vi "BotSpeak_HTTP.vi"(0 "BotSpeak File Name":path, 1 "URL":string, 2 "BotSpeak Code":string, 3 "cookie file":path) -> (7 "connection\nerror":errorcluster, 8 "file error":errorcluster)   [LabVIEW 2014]
uses:
  <vilib>/httpClient/POSTFile.vi
  <vilib>/httpClient/LabVIEWHTTPClient.lvlib
panel:
  # "Macintosh HD:Users:gabbyvukasin:Documents:Tufts:Independent Study:EV3Server:BotSpeakCode.txt"
  # "Macintosh HD:Users:gabbyvukasin:Documents:Tufts:Independent Study:EV3Server:cookies.txt"
  # "SET DIO[1],1"
  # "192.168.2.3:2012"
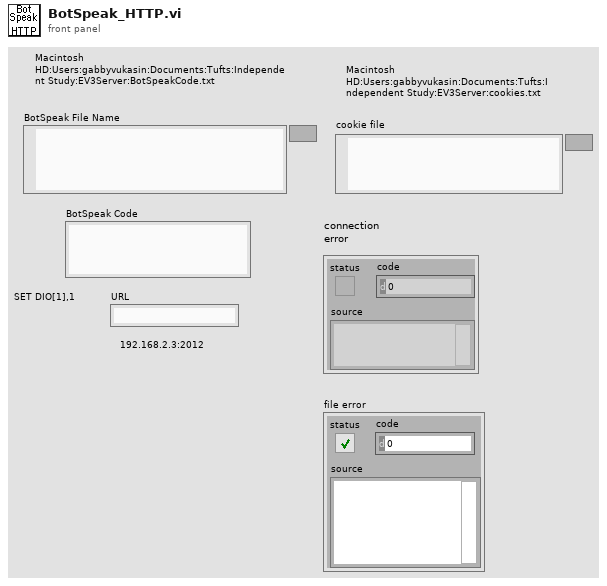
[diagram p1: front panel]
types:
  T1 = typedef "LabVIEWHTTPClient.lvlib/ClientHandle.ctl" = refnum<k1>
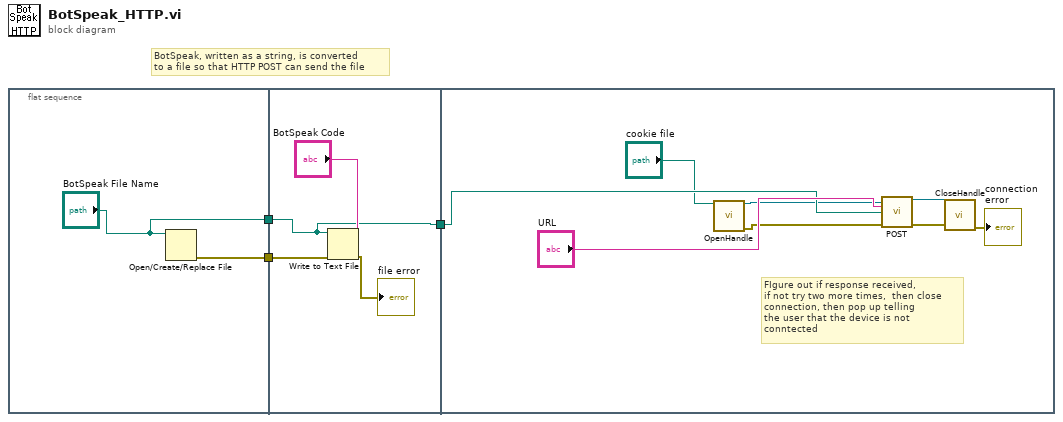
[diagram p0: block diagram]
diagram:
  # "BotSpeak, written as a string, is converted\nto a file so that HTTP POST can send the file"
  n1 = flat-sequence {
    tunnel: ["BotSpeak File Name"] -> w2
    tunnel: [w5] -> w1
    tunnel: [w6] -> w3
    tunnel: w2 -> [w6]
    tunnel: w1 -> [w8]
    tunnel: w3 -> [w14]
    frame #0 {
      n2 = Open/Create/Replace File(file path (use dialog)="BotSpeak File Name") -> (error out=w5:errorcluster)  [unwired: 5 in, 2 out]
    }
    frame #1 {
      n3 = Write to Text File(file (use dialog)=w6, text="BotSpeak Code", error in=w8) -> (error out=→"file error":errorcluster)  [unwired: 1 in, 2 out]
    }
    frame #2 {
      # "FIgure out if response received, \nif not try two more times,  then close \nconnection, then pop up telling\nthe user that the device is not \nconntected"
      n4 = call <vilib>:"OpenHandle.vi"("cookie file"="cookie file") -> ("client handle out"=w13:T1, "error out"=w12:errorcluster)  [unwired: 13 in]
      n5 = call-poly <vilib>:"POST.vi"("client handle"=w13, "url"="URL", "file"=w14, "error in (no error)"=w12) -> ("client handle out"=w11:T1, "error out"=w15:errorcluster)  [unwired: 8 in, 2 out]
      n6 = call <vilib>:"CloseHandle.vi"("client handle"=w11, "error in (no error)"=w15) -> ("error out"=→"connection\nerror":errorcluster)  [unwired: 13 in]
    }
  }
